vi "Chopper Motor Test.vi"(7 "Measurement Started?":bool, 8 "error in (no error)":errorcluster, 11 "Session Handle in":T1) -> (0 "error out":errorcluster, 2 "Passed?":bool, 3 "Session Handle out":T1 caption="Gas")   [LabVIEW 2015, in "PAS.lvclass"]
uses:
  PAS.lvclass
  Typedefs/Session Handle.ctl
panel:
  out "Frequency":dbl
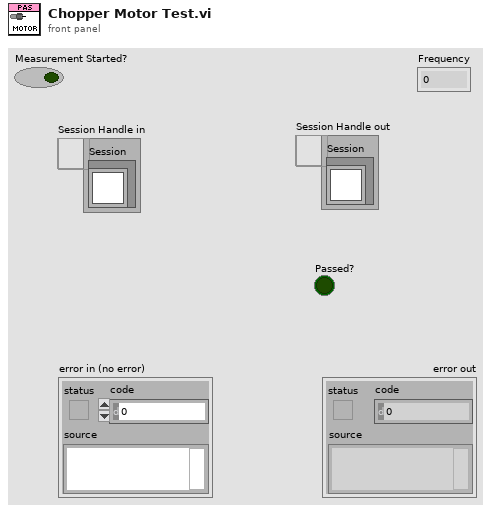
[diagram p1: front panel]
types:
  T1 = typedef "PAS.lvclass/Session Handle.ctl" = refnum<data-value>
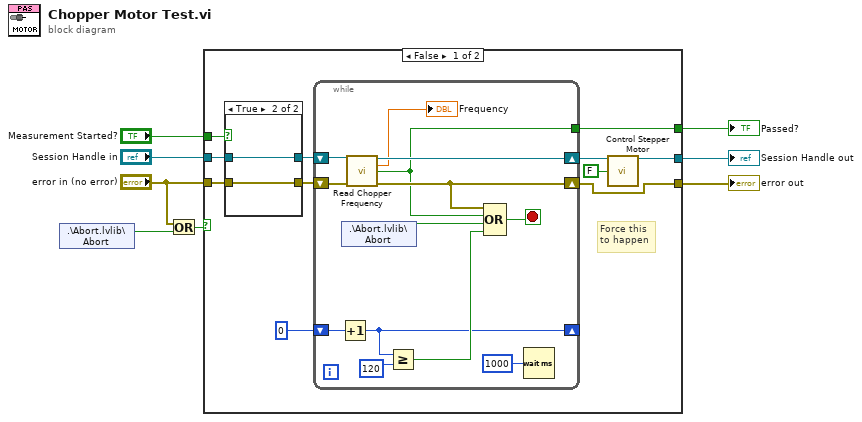
[diagram p0: block diagram]
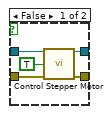
[diagram p2: hidden frame]
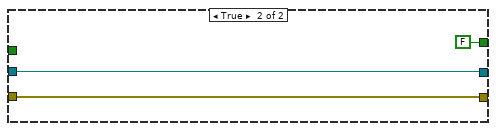
[diagram p3: hidden frame]
diagram:
  n1 = shared-variable ".\\Abort.lvlib\\Abort"() -> (w3:bool)  [unwired: 1 in, 1 out]
  n2 = Or(x="error in (no error)", y=w3) -> (x .or. y?=w2:bool)
  n3 = case shown="False" w2 {
    tunnel: [w17 w40] -> w8
    tunnel: "Session Handle in" -> [w16 w41]
    tunnel: "error in (no error)" -> [w15 w40]
    tunnel: [w14 FALSE ("Finished Ramping?")] -> w6
    tunnel: [w11 w41] -> w5
    tunnel: "Measurement Started?" -> [w9 _]
    frame False {
      # "Force this\nto happen"
      n4 = case shown="True" w9 {
        tunnel: [w24 w26] -> w19
        tunnel: [w23 w25] -> w18
        tunnel: w16 -> [w22 w26]
        tunnel: w15 -> [w21 w25]
        frame False {
          n5 = call "Control Stepper Motor.vi"("Session Handle in"=w22, "Start?"=TRUE, "error in (no error)"=w21) -> ("Session Handle out"=w24:T1, "error out"=w23:errorcluster)  [unwired: 10 in, 1 out]
        }
        frame True {
        }
      }
      n6 = while {
        shift-right: [w35] -> w17
        shift-left: w18 -> [w38]
        shift-right: [w37] -> w12
        shift-left: w19 -> [w39]
        tunnel: [w33] -> w14
        shift-right: [w29] -> _
        shift-left: u32 0 ("milliseconds to wait") -> [w32]
        stop <- w34 stop-if-true
        n7 = Increment(x=w32) -> (x+1=w29:u32)
        n8 = shared-variable ".\\Abort.lvlib\\Abort"() -> (w27:bool)  [unwired: 1 in, 1 out]
        n9 = call "Read Chopper Frequency.vi"("Session Handle in"=w39, "error in (no error)"=w38) -> ("Session Handle out"=w37:T1, "Frequency"=→"Frequency":dbl, "Finished Ramping?"=w33:bool, "error out"=w35:errorcluster)  [unwired: 9 in, 1 out]
        n10 = Greater Or Equal?(x=w29, y=u32 120) -> (x >= y?=w30:bool)
        n11 = Compound Arithmetic op=OR(w35, w33, w27, w30) -> (w34:bool)
        n12 = Wait (ms)(milliseconds to wait=u32 1000) -> ()  [unwired: 1 out]
      }
      n13 = call "Control Stepper Motor.vi"("Session Handle in"=w12, "Start?"=FALSE) -> ("Session Handle out"=w11:T1)  [unwired: 11 in, 2 out]
    }
    frame True {
    }
  }
  "error out" <- w8
  "Passed?" <- w6
  "Session Handle out" <- w5
